vi "Retrieve Occupancy Grid.vi"(1 "Robot X":i32, 2 "Robot Y":i32, 3 "Col":i32, 4 "Row":i32) -> (0 "element":dbl)   [LabVIEW 2009]
panel:
  in  "Occupancy Grid":dbl[][](array[numeric])
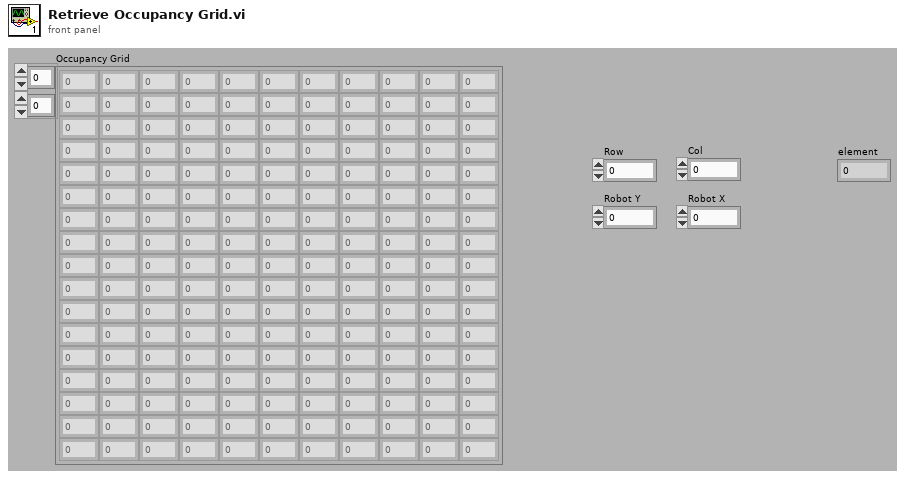
[diagram p1: front panel]
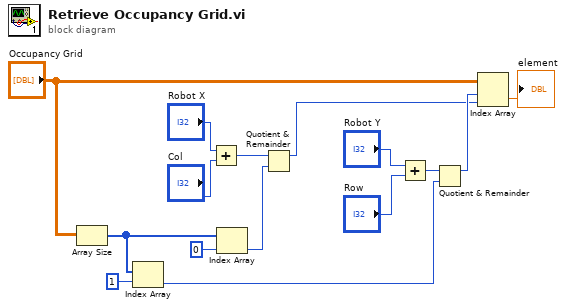
[diagram p0: block diagram]
diagram:
  n1 = Array Size(array="Occupancy Grid") -> (size(s)=w6:i32[])
  n2 = Index Array(array=w6, index=1) -> (element=w4:i32)
  n3 = Add(x="Robot X", y="Col") -> (x+y=w10:i32)
  n4 = Index Array(array=w6, index=0) -> (element=w5:i32)
  n5 = Quotient & Remainder(x=w10, y=w5) -> (x-y*floor(x/y)=w1:i32)  [unwired: 1 out]
  n6 = Add(x="Robot Y", y="Row") -> (x+y=w9:i32)
  n7 = Quotient & Remainder(x=w9, y=w4) -> (x-y*floor(x/y)=w2:i32)  [unwired: 1 out]
  n8 = Index Array(array="Occupancy Grid", index (row)=w2, index (col)=w1) -> (element=→"element":dbl)
